vi "mover.vi"() -> ()   [LabVIEW 2024]
uses:
  Sub_Vis/Operations.ctl
  Sub_Vis/truePosition.vi
panel:
  in  "Wrtie current data to file":bool
  in  "Scanning Mode":enum32{"Automatic"}(tab)
  out "Scan Progress":dbl(slide) scale=0.0..1.0
  in  "Small Step Distance (microns)":dbl format="%#_13g"
  in  "Number Of Small Steps":i32
  in  "Number of Large Steps":i32
  in  "Large Step Distance (microns)":dbl format="%#_13g"
  in  "Abort":bool
  in  "Change File":bool
  out "Operation":T1=enum."Nothing"
  out "stored counts":dbl[unit][](array[numeric])
  out "stored positions":dbl[](array[numeric])
  in  "End":bool
  out "error out 20":errorcluster
  out "error out 6":errorcluster
  out "error out 21":errorcluster
  out "error out 16":errorcluster
  in  "Hardware Limit (mm)":dbl=100.0 format="%#_13g"
  out "error out 15":errorcluster
  out "error out 14":errorcluster
  out "error out 10":errorcluster
  in  "Home":bool
  out "error out 9":errorcluster
  out "True Position (number)":dbl[unit] format="%#_10f"
  in  "error in 4":errorcluster
  out "error out 13":errorcluster
  out "error out 12":errorcluster
  in  "Target Position (mm)":dbl format="%#_13g"
  out "error out 11":errorcluster
  in  "Go To Position":bool
  out "error out 5":errorcluster
  in  "Advance Step":bool
  out "True Position":ext(slide) scale=0.0..25.0
  out "error out 3":errorcluster
  in  "Axis #":i32=1
  in  "Port #":i32=3
  in  "Step Distance (microns)":dbl format="%#_13g"
  out "error out 2":errorcluster
  # "Movement Controls"
  # "Configuration"
  # "Counter"
  # "Motor"
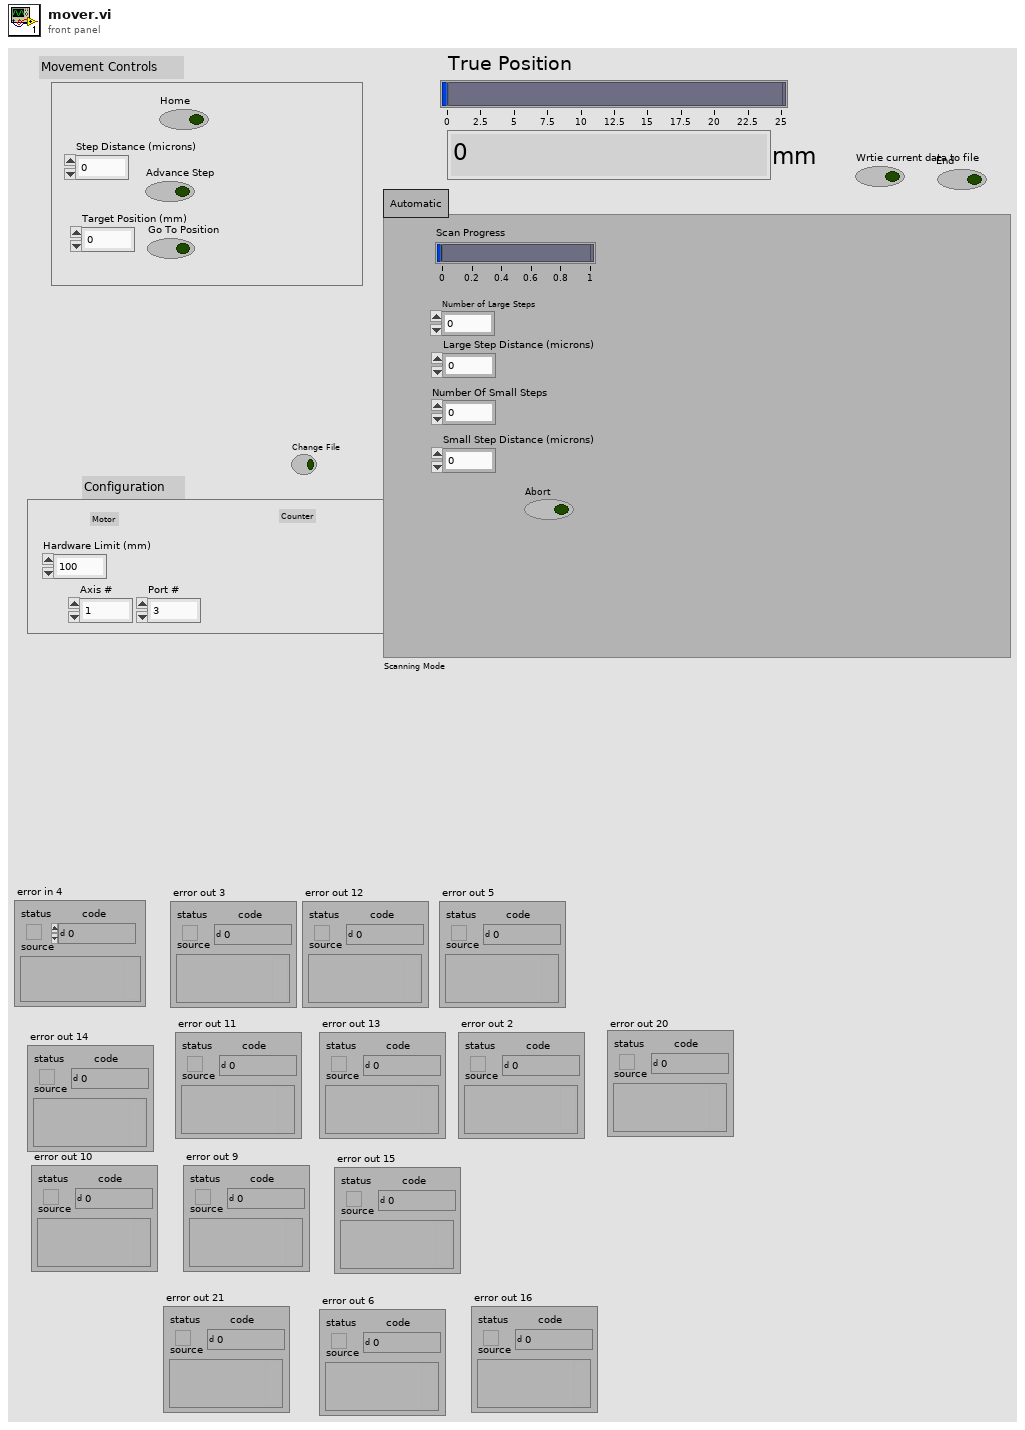
[diagram p1: front panel]
types:
  T1 = typedef "Operations.ctl" = enum16{"Home", "Go To Position", "Advance Step", "Scan", "Write to File", "Change File", "End", "Nothing"}
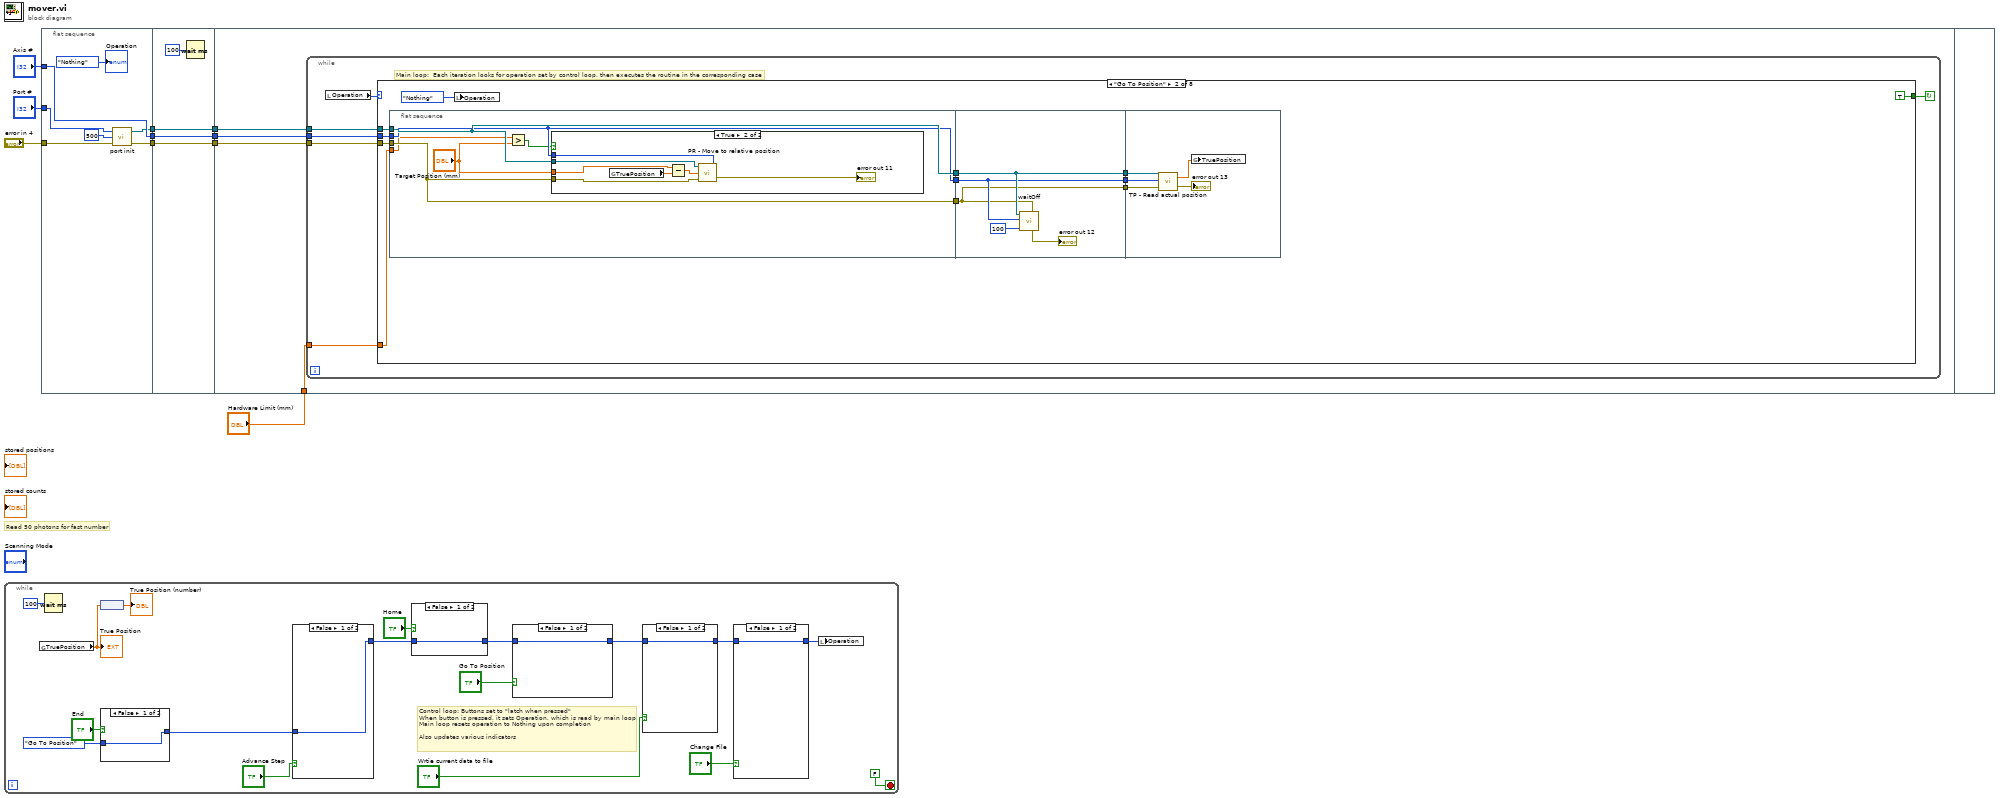
[diagram p0: block diagram]
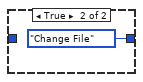
[diagram p2: hidden frame]
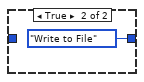
[diagram p3: hidden frame]
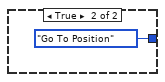
[diagram p4: hidden frame]
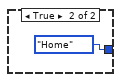
[diagram p5: hidden frame]
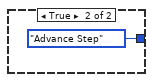
[diagram p6: hidden frame]
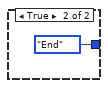
[diagram p7: hidden frame]
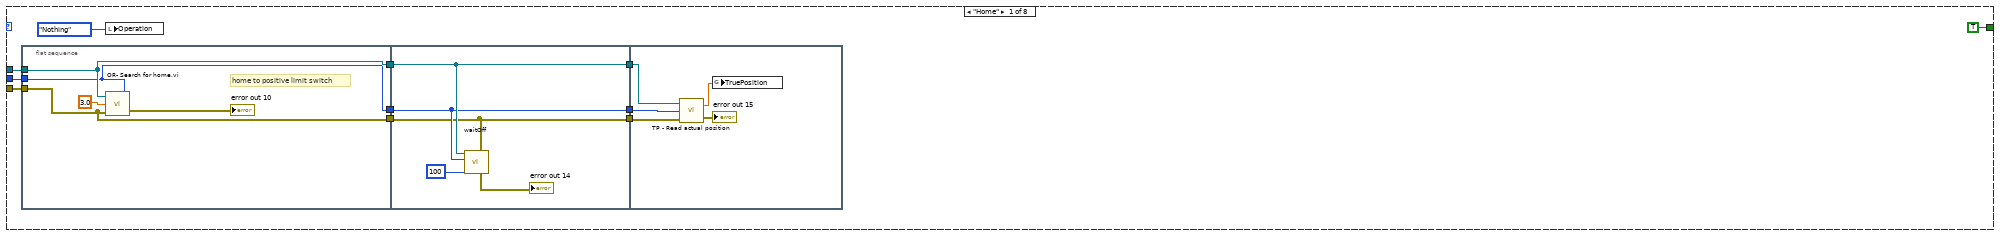
[diagram p8: hidden frame]
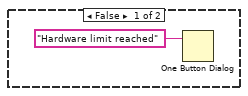
[diagram p9: hidden frame]
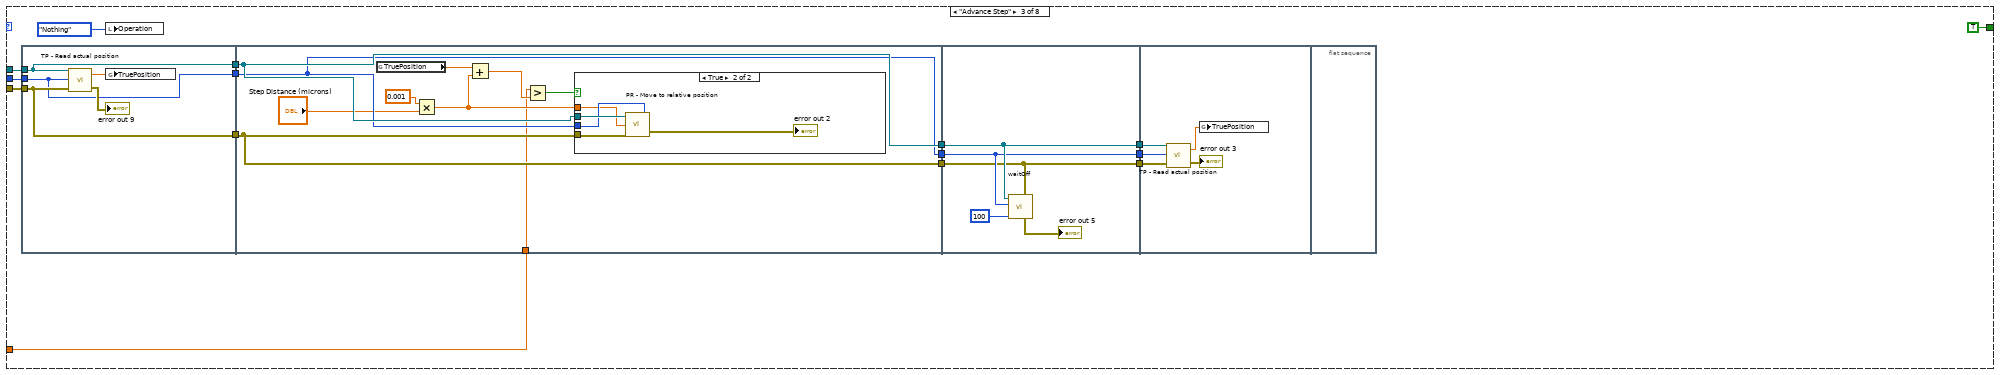
[diagram p10: hidden frame]
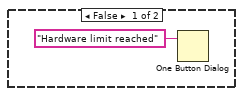
[diagram p11: hidden frame]
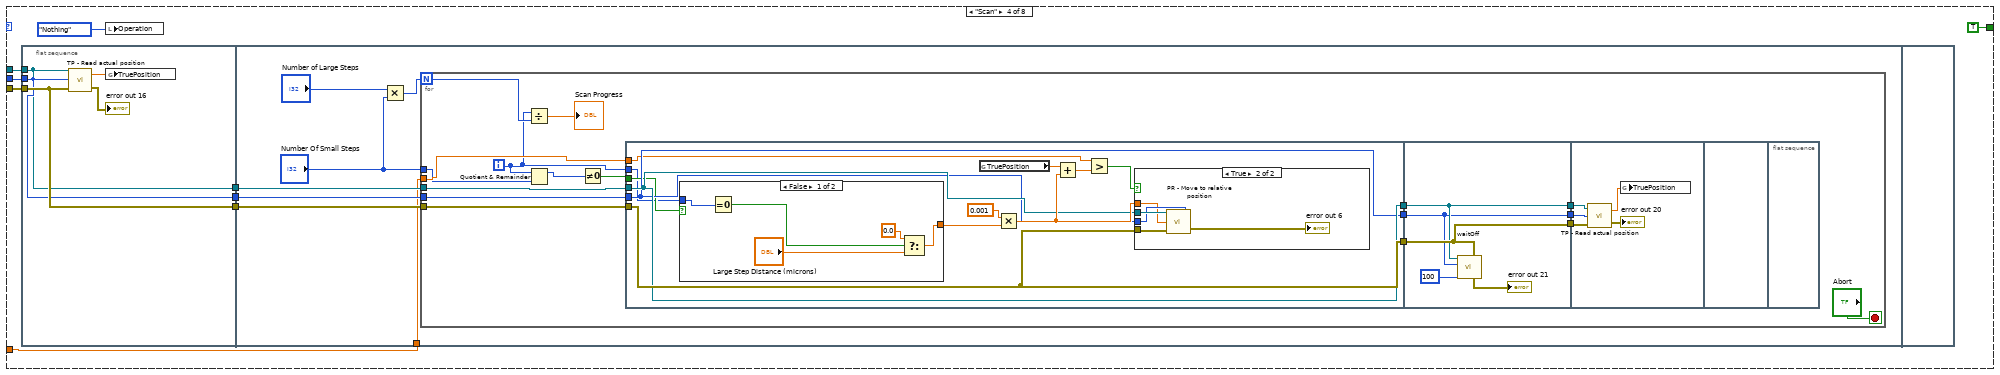
[diagram p12: hidden frame]
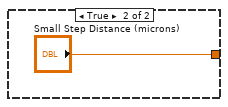
[diagram p13: hidden frame]
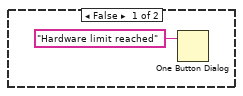
[diagram p14: hidden frame]
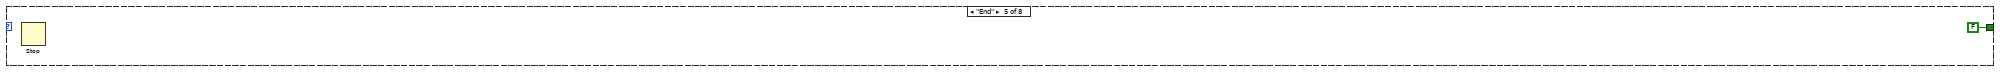
[diagram p15: hidden frame]
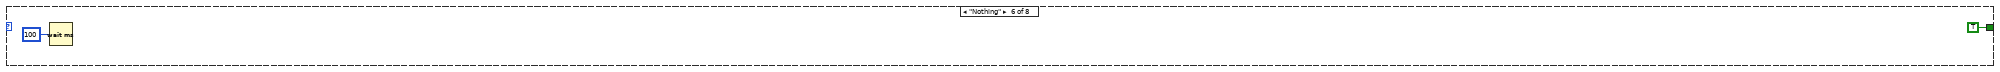
[diagram p16: hidden frame]
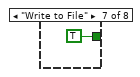
[diagram p17: hidden frame]
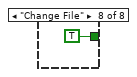
[diagram p18: hidden frame]
diagram:
  # "Read 50 photons for fast number"
  n1 = while {
    stop <- FALSE stop-if-true
    # "Control loop: Buttons set to \"latch when pressed\"\nWhen button is pressed, it sets Operation, which is read by main loop\nMain loop resets operation to Nothing upon completion\n\nAlso updates various indicators"
    n2 = global read "truePosition.vi" "TruePosition"() -> (w25:dbl)
    "True Position" <- w25
    n3 = Wait (ms)(milliseconds to wait=100) -> ()  [unwired: 1 out]
    n4 = node(w25) -> (→"True Position (number)":dbl[unit])
    n5 = case shown="False" "End" {
      tunnel: [w38 Operations."End"] -> w11
      tunnel: Operations."Go To Position" -> [w38 _]
      frame False {
      }
      frame True {
      }
    }
    n6 = case shown="False" "Advance Step" {
      tunnel: [w36 Operations."Advance Step"] -> w17
      tunnel: w11 -> [w36 _]
      frame False {
      }
      frame True {
      }
    }
    n7 = case shown="False" "Home" {
      tunnel: [w34 Operations."Home"] -> w18
      tunnel: w17 -> [w34 _]
      frame False {
      }
      frame True {
      }
    }
    n8 = case shown="False" "Go To Position" {
      tunnel: w18 -> [w32 _]
      tunnel: [w32 Operations."Go To Position"] -> w16
      frame False {
      }
      frame True {
      }
    }
    n9 = case shown="False" "Wrtie current data to file" {
      tunnel: w16 -> [w30 _]
      tunnel: [w30 Operations."Write to File"] -> w13
      frame False {
      }
      frame True {
      }
    }
    n10 = case shown="False" "Change File" {
      tunnel: w13 -> [w28 _]
      tunnel: [w28 Operations."Change File"] -> w12
      frame False {
      }
      frame True {
      }
    }
    n11 = local write "Operation"(w12) -> ()
  }
  n12 = flat-sequence {
    tunnel: "error in 4" -> [w42]
    tunnel: "Axis #" -> [w46]
    tunnel: "Port #" -> [w44]
    tunnel: [w40] -> w8
    tunnel: [w46] -> w6
    tunnel: [w41] -> w4
    tunnel: w8 -> [w50]
    tunnel: [w50] -> w7
    tunnel: w6 -> [w49]
    tunnel: [w49] -> w5
    tunnel: w4 -> [w48]
    tunnel: [w48] -> w3
    tunnel: w7 -> [w54]
    tunnel: w5 -> [w53]
    tunnel: w3 -> [w52]
    tunnel: "Hardware Limit (mm)" -> [w51]
    frame #0 {
      n13 = call "port init.vi"("error in"=w42, "Timeout (ms)"=500, "SerialPort"=w44) -> ("error out"=w41:errorcluster, "Visa Handle"=w40:refnum<visa-resource-name>)  [unwired: 1 in]
      "Operation" <- Operations."Nothing"
    }
    frame #1 {
      n14 = Wait (ms)(milliseconds to wait=100) -> ()  [unwired: 1 out]
    }
    frame #2 {
      n15 = while {
        tunnel: w54 -> [w56]
        tunnel: w53 -> [w59]
        tunnel: w52 -> [w58]
        tunnel: w51 -> [w57]
        stop <- w55 continue-if-true
        # "Main loop:  Each iteration looks for operation set by control loop, then executes the routine in the corresponding case"
        n16 = local read "Operation"() -> (w60:T1)
        n17 = case shown="\"Go To Position\"" w60 {
          tunnel: w56 -> [w69 w96 w137 w177 _ _ _ _]
          tunnel: w59 -> [w68 w95 w136 w176 _ _ _ _]
          tunnel: w58 -> [w67 w97 w135 w175 _ _ _ _]
          tunnel: w57 -> [_ w98 w134 w171 _ _ _ _]
          tunnel: [TRUE TRUE TRUE TRUE FALSE TRUE TRUE TRUE] -> w55
          frame "Home" {
            n18 = flat-sequence {
              tunnel: w69 -> [w74]
              tunnel: w68 -> [w73]
              tunnel: w67 -> [w72]
              tunnel: [w74] -> w66
              tunnel: [w73] -> w65
              tunnel: [w72] -> w64
              tunnel: w66 -> [w79]
              tunnel: w65 -> [w78]
              tunnel: w64 -> [w77]
              tunnel: [w79] -> w63
              tunnel: [w78] -> w62
              tunnel: [w77] -> w61
              tunnel: w63 -> [w84]
              tunnel: w62 -> [w83]
              tunnel: w61 -> [w82]
              frame #0 {
                # "home to positive limit switch"
                n19 = call "OR- Search for home,vi"("Axis  #"=w73, "error in"=w72, "Home mode"=3.0, "VISA handle in"=w74) -> ("error out"=→"error out 10":errorcluster)
              }
              frame #1 {
                n20 = call "waitOff.vi"("error in"=w77, "queueing interval"=100, "Axis #"=w78, "VISA handle in"=w79) -> ("error out 2"=→"error out 14":errorcluster)  [unwired: 7 in]
              }
              frame #2 {
                n21 = call "TP - Read actual position.vi"("error in"=w82, "Axis"=w83, "VISA handle in"=w84) -> ("error out"=→"error out 15":errorcluster, "Query the current actual\nposition - read"=w85:dbl)
                n22 = global write "truePosition.vi" "TruePosition"(w85) -> ()
              }
            }
            n23 = local write "Operation"(Operations."Nothing") -> ()
          }
          frame "Go To Position" {
            n24 = flat-sequence {
              tunnel: [w102] -> w92
              tunnel: [w104] -> w91
              tunnel: [w103] -> w90
              tunnel: w96 -> [w104]
              tunnel: w95 -> [w103]
              tunnel: w97 -> [w102]
              tunnel: w98 -> [w99]
              tunnel: [w114] -> w89
              tunnel: w92 -> [w114]
              tunnel: [w116] -> w88
              tunnel: w91 -> [w116]
              tunnel: [w115] -> w87
              tunnel: w90 -> [w115]
              tunnel: w89 -> [w122]
              tunnel: w88 -> [w120]
              tunnel: w87 -> [w119]
              frame #0 {
                n25 = Greater?(x=w99, y="Target Position (mm)") -> (0:w100:bool)
                n26 = case shown="True" w100 {
                  tunnel: "Target Position (mm)" -> [_ w108]
                  tunnel: w104 -> [_ w111]
                  tunnel: w103 -> [_ w110]
                  tunnel: w102 -> [_ w109]
                  frame False {
                    n27 = One Button Dialog(message="Hardware limit reached") -> ()  [unwired: 1 in, 1 out]
                  }
                  frame True {
                    n28 = global read "truePosition.vi" "TruePosition"() -> (w107:dbl)
                    n29 = Subtract(x=w108, y=w107) -> (x-y=w106:dbl)
                    n30 = call "PR - Move to relative position.vi"("Axis  #"=w110, "error in"=w109, "Relative motion increment"=w106, "VISA handle in"=w111) -> ("error out"=→"error out 11":errorcluster)
                  }
                }
              }
              frame #1 {
                n31 = call "waitOff.vi"("error in"=w114, "queueing interval"=100, "Axis #"=w115, "VISA handle in"=w116) -> ("error out 2"=→"error out 12":errorcluster)  [unwired: 7 in]
              }
              frame #2 {
                n32 = call "TP - Read actual position.vi"("error in"=w122, "Axis"=w119, "VISA handle in"=w120) -> ("error out"=→"error out 13":errorcluster, "Query the current actual\nposition - read"=w118:dbl)
                n33 = global write "truePosition.vi" "TruePosition"(w118) -> ()
              }
            }
            n34 = local write "Operation"(Operations."Nothing") -> ()
          }
          frame "Advance Step" {
            n35 = flat-sequence {
              tunnel: w135 -> [w141]
              tunnel: w136 -> [w140]
              tunnel: w137 -> [w139]
              tunnel: [w139] -> w131
              tunnel: [w140] -> w130
              tunnel: [w141] -> w129
              tunnel: [w150] -> w128
              tunnel: [w152] -> w127
              tunnel: [w151] -> w126
              tunnel: w131 -> [w152]
              tunnel: w130 -> [w151]
              tunnel: w129 -> [w150]
              tunnel: w134 -> [w145]
              tunnel: [w160] -> w125
              tunnel: w128 -> [w160]
              tunnel: [w162] -> w124
              tunnel: w127 -> [w162]
              tunnel: [w161] -> w123
              tunnel: w126 -> [w161]
              tunnel: w125 -> [w168]
              tunnel: w124 -> [w166]
              tunnel: w123 -> [w165]
              frame #0 {
                n36 = call "TP - Read actual position.vi"("error in"=w141, "Axis"=w140, "VISA handle in"=w139) -> ("error out"=→"error out 9":errorcluster, "Query the current actual\nposition - read"=w138:dbl)
                n37 = global write "truePosition.vi" "TruePosition"(w138) -> ()
              }
              frame #1 {
                n38 = global read "truePosition.vi" "TruePosition"() -> (w143:dbl)
                n39 = Multiply(x=0.001, y="Step Distance (microns)") -> (x*y=w147:dbl)
                n40 = Add(x=w143, y=w147) -> (x+y=w146:dbl)
                n41 = Greater?(x=w145, y=w146) -> (0:w144:bool)
                n42 = case shown="True" w144 {
                  tunnel: w152 -> [_ w157]
                  tunnel: w151 -> [_ w156]
                  tunnel: w150 -> [_ w155]
                  tunnel: w147 -> [_ w154]
                  frame False {
                    n43 = One Button Dialog(message="Hardware limit reached") -> ()  [unwired: 1 in, 1 out]
                  }
                  frame True {
                    n44 = call "PR - Move to relative position.vi"("Axis  #"=w156, "error in"=w155, "Relative motion increment"=w154, "VISA handle in"=w157) -> ("error out"=→"error out 2":errorcluster)
                  }
                }
              }
              frame #2 {
                n45 = call "waitOff.vi"("error in"=w160, "queueing interval"=100, "Axis #"=w161, "VISA handle in"=w162) -> ("error out 2"=→"error out 5":errorcluster)  [unwired: 7 in]
              }
              frame #3 {
                n46 = call "TP - Read actual position.vi"("error in"=w168, "Axis"=w165, "VISA handle in"=w166) -> ("error out"=→"error out 3":errorcluster, "Query the current actual\nposition - read"=w164:dbl)
                n47 = global write "truePosition.vi" "TruePosition"(w164) -> ()
              }
              frame #4 {
              }
            }
            n48 = local write "Operation"(Operations."Nothing") -> ()
          }
          frame "Scan" {
            n49 = flat-sequence {
              tunnel: w175 -> [w181]
              tunnel: w176 -> [w180]
              tunnel: w177 -> [w179]
              tunnel: [w179] -> w174
              tunnel: [w180] -> w173
              tunnel: [w181] -> w172
              tunnel: w174 -> [w188]
              tunnel: w173 -> [w187]
              tunnel: w172 -> [w189]
              tunnel: w171 -> [w186]
              frame #0 {
                n50 = call "TP - Read actual position.vi"("error in"=w181, "Axis"=w180, "VISA handle in"=w179) -> ("error out"=→"error out 16":errorcluster, "Query the current actual\nposition - read"=w178:dbl)
                n51 = global write "truePosition.vi" "TruePosition"(w178) -> ()
              }
              frame #1 {
                n52 = Multiply(x="Number of Large Steps", y="Number Of Small Steps") -> (x*y=w185:i32)
                n53 = for {
                  N: w185 -> [w195]
                  tunnel: w189 -> [w200]
                  tunnel: w188 -> [w199]
                  tunnel: w187 -> [w198]
                  tunnel: w186 -> [w197]
                  tunnel: "Number Of Small Steps" -> [w194]
                  i -> [w190]
                  stop <- "Abort" stop-if-true
                  n54 = Divide(x=w190, y=w195) -> (x/y=→"Scan Progress":dbl)
                  n55 = Quotient & Remainder(x=w190, y=w194) -> (x-y*floor(x/y)=w193:i32)  [unwired: 1 out]
                  n56 = Not Equal To 0?(x=w193) -> (x != 0?=w192:bool)
                  n57 = flat-sequence {
                    tunnel: [w211] -> w206
                    tunnel: [w210] -> w205
                    tunnel: [w212] -> w204
                    tunnel: w200 -> [w212]
                    tunnel: w199 -> [w211]
                    tunnel: w198 -> [w210]
                    tunnel: w197 -> [w209]
                    tunnel: w192 -> [w208]
                    tunnel: w190 -> [w207]
                    tunnel: w206 -> [w232]
                    tunnel: w205 -> [w231]
                    tunnel: w204 -> [w233]
                    tunnel: [w233] -> w203
                    tunnel: [w232] -> w202
                    tunnel: [w231] -> w201
                    tunnel: w203 -> [w239]
                    tunnel: w202 -> [w238]
                    tunnel: w201 -> [w237]
                    frame #0 {
                      n58 = case shown="False" w208 {
                        tunnel: [w222 "Small Step Distance (microns)"] -> w218
                        tunnel: w207 -> [w219 _]
                        frame False {
                          n59 = Equal To 0?(x=w219) -> (x = 0?=w220:bool)
                          n60 = Select(t=0.0, s=w220, f="Large Step Distance (microns)") -> (s? t:f=w222:dbl)
                        }
                        frame True {
                        }
                      }
                      n61 = global read "truePosition.vi" "TruePosition"() -> (w213:dbl)
                      n62 = Multiply(x=0.001, y=w218) -> (x*y=w216:dbl)
                      n63 = Add(x=w213, y=w216) -> (x+y=w215:dbl)
                      n64 = Greater?(x=w209, y=w215) -> (0:w214:bool)
                      n65 = case shown="True" w214 {
                        tunnel: w211 -> [_ w229]
                        tunnel: w210 -> [_ w228]
                        tunnel: w212 -> [_ w227]
                        tunnel: w216 -> [_ w226]
                        frame False {
                          n66 = One Button Dialog(message="Hardware limit reached") -> ()  [unwired: 1 in, 1 out]
                        }
                        frame True {
                          n67 = call "PR - Move to relative position.vi"("Axis  #"=w228, "error in"=w227, "Relative motion increment"=w226, "VISA handle in"=w229) -> ("error out"=→"error out 6":errorcluster)
                        }
                      }
                    }
                    frame #1 {
                      n68 = call "waitOff.vi"("error in"=w233, "queueing interval"=100, "Axis #"=w231, "VISA handle in"=w232) -> ("error out 2"=→"error out 21":errorcluster)  [unwired: 7 in]
                    }
                    frame #2 {
                      n69 = call "TP - Read actual position.vi"("error in"=w239, "Axis"=w237, "VISA handle in"=w238) -> ("error out"=→"error out 20":errorcluster, "Query the current actual\nposition - read"=w236:dbl)
                      n70 = global write "truePosition.vi" "TruePosition"(w236) -> ()
                    }
                    frame #3 {
                    }
                    frame #4 {
                    }
                  }
                }
              }
              frame #2 {
              }
            }
            n71 = local write "Operation"(Operations."Nothing") -> ()
          }
          frame "End" {
            n72 = Stop() -> ()  [unwired: 1 in]
          }
          frame "Nothing" {
            n73 = Wait (ms)(milliseconds to wait=u32 100) -> ()  [unwired: 1 out]
          }
          frame "Write to File" {
          }
          frame "Change File" {
          }
        }
      }
    }
    frame #3 {
    }
  }
